vi "CleanUp.vi"(0 "object in":refnum<class "KickTo.lvclass">, 5 "error in (no error)":errorcluster) -> (14 "object out":refnum<class "KickTo.lvclass">, 19 "error out":errorcluster)   [LabVIEW 2022 SP3, in "KickTo.lvclass"]
uses:
  KickTo.lvclass
  KickTo.lvclass/KickTo.ctl
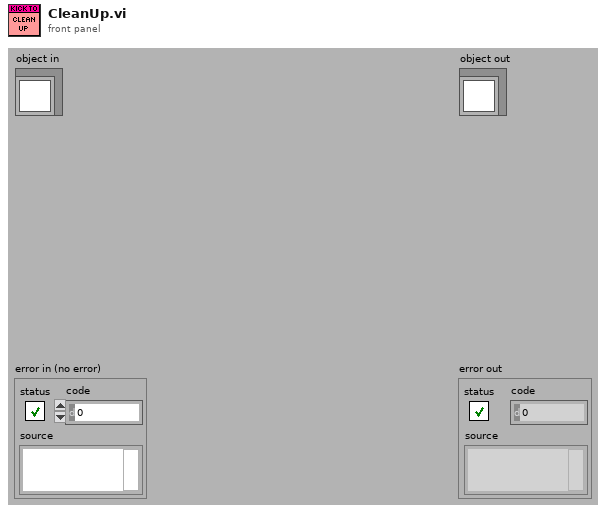
[diagram p1: front panel]
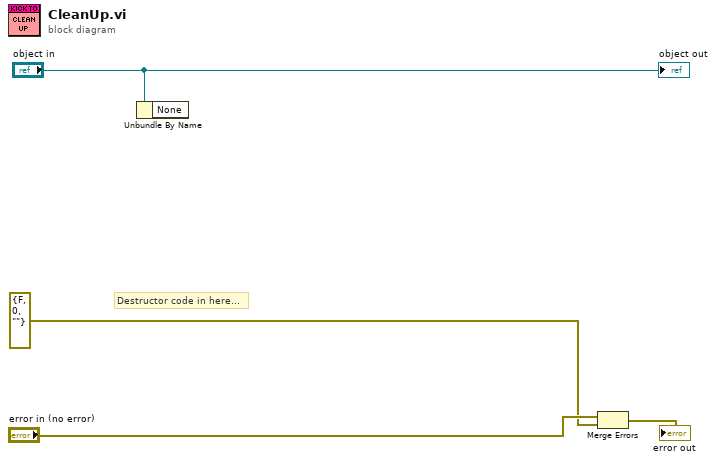
[diagram p0: block diagram]
diagram:
  # "Destructor code in here..."
  n1 = Unbundle By Name("object in") -> ()  [unwired: 1 out]
  n2 = Merge Errors("error in (no error)", errorcluster {"status"=FALSE, "code"=0, "source"=""} ("error in (no error)")) -> (→"error out":errorcluster)
  "object out" <- "object in"
